vi "Write target.vi"(8 "error in (no error)":errorcluster, 10 "target":i32, 11 "SecMirror in":refnum<class "SecMirror.lvclass">) -> (0 "error out":errorcluster, 3 "SecMirror out":refnum<class "SecMirror.lvclass">)   [LabVIEW 2018, in "SecMirror.lvclass"]
uses:
  SecMirror.lvclass
  SecMirror.lvclass/SecMirror.ctl
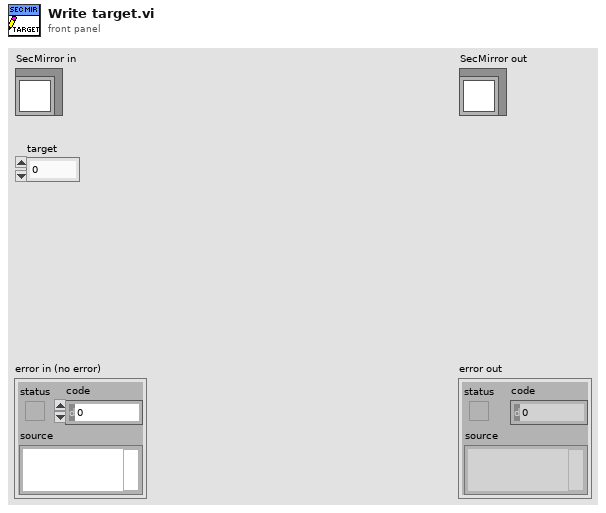
[diagram p1: front panel]
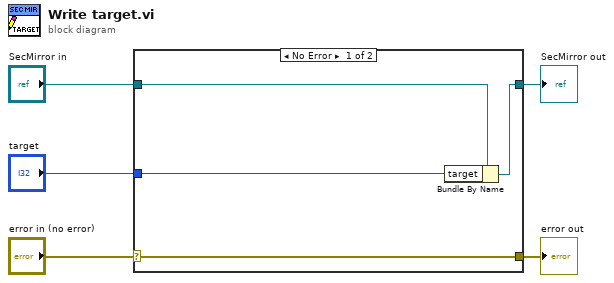
[diagram p0: block diagram]
diagram:
  n1 = case shown="No Error" "error in (no error)" {
    selector: "error in (no error)" -> [w9 w10]
    tunnel: [w9 w10] -> w4
    tunnel: [w7 w11] -> w2
    tunnel: "SecMirror in" -> [w8 w11]
    tunnel: "target" -> [w6 _]
    frame No Error {
      n2 = Bundle By Name(cluster=w8, "target"=w6) -> (w7:refnum<class "SecMirror.lvclass">)
    }
    frame Error {
    }
  }
  "error out" <- w4
  "SecMirror out" <- w2
